vi "VI Tree.vi"   [LabVIEW 2013]
uses:
  Utility/Get Step Address(AC Program).vi
  Configure/Write Step Data(AC Program).vi
  Data/Read Step Data(AC Program).vi
  Action/TEST(Program Mode).vi
  Action/Reset(Program Mode).vi
panel:
  # "(c) 2017 Preen AC Source Interument.  ALL RIGHTS RESERVED."
  # "SEE DIAGRAM\nFOR VI TREE."
  # "Version 1.00"
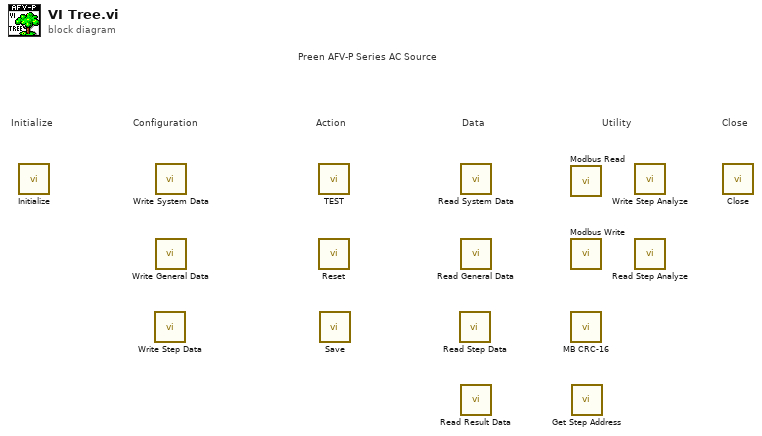
[diagram p0: block diagram]
diagram:
  # "Preen AFV-P Series AC Source"
  # "Configuration"
  # "Utility"
  # "Data"
  # "Action"
  # "Close"
  # "Initialize"
  n1 = call "Initialize.vi"() -> ()  [unwired: 10 in, 2 out]
  n2 = call-poly "Write Step Data.vi"() -> ()  [unwired: 10 in, 2 out]
  n3 = call "Write System Data.vi"() -> ()  [unwired: 10 in, 2 out]
  n4 = call "Write General Data.vi"() -> ()  [unwired: 10 in, 2 out]
  n5 = call-poly "TEST.vi"() -> ()  [unwired: 10 in, 2 out]
  n6 = call-poly "Reset.vi"() -> ()  [unwired: 10 in, 2 out]
  n7 = call "Save.vi"() -> ()  [unwired: 10 in, 2 out]
  n8 = call-poly "Read Step Data.vi"() -> ()  [unwired: 9 in, 3 out]
  n9 = call "Read System Data.vi"() -> ()  [unwired: 9 in, 3 out]
  n10 = call "Read General Data.vi"() -> ()  [unwired: 9 in, 3 out]
  n11 = call "Read Result Data.vi"() -> ()  [unwired: 9 in, 3 out]
  n12 = call "Modbus Read.vi"() -> ()  [unwired: 9 in, 3 out]
  n13 = call "Modbus Write.vi"() -> ()  [unwired: 10 in, 2 out]
  n14 = call "MB CRC-16.vi"() -> ()  [unwired: 9 in, 3 out]
  n15 = call-poly "Get Step Address.vi"() -> ()  [unwired: 6 in, 6 out]
  n16 = call "Write Step Analyze.vi"() -> ()  [unwired: 11 in, 1 out]
  n17 = call "Read Step Analyze.vi"() -> ()  [unwired: 11 in, 1 out]
  n18 = call "Close.vi"() -> ()  [unwired: 11 in, 1 out]
